vi "Read sequencia_ant.vi"(8 "error in (no error)":errorcluster, 11 "Opt_Selector in":refnum<class "Opt_Selector.lvclass">) -> (0 "error out":errorcluster, 2 "sequencia_ant":u16, 3 "Opt_Selector out":refnum<class "Opt_Selector.lvclass">)   [LabVIEW 2018, in "Opt_Selector.lvclass"]
uses:
  Opt_Selector.lvclass
  Opt_Selector.lvclass/Opt_Selector.ctl
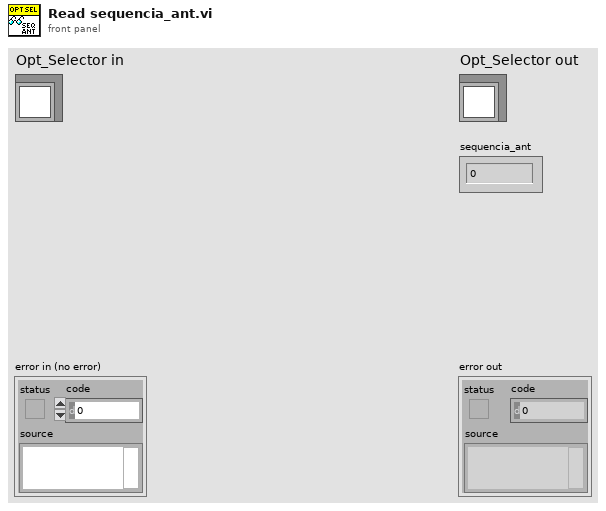
[diagram p1: front panel]
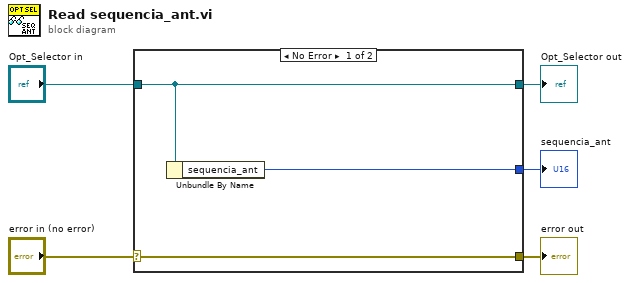
[diagram p0: block diagram]
diagram:
  n1 = case shown="No Error" "error in (no error)" {
    selector: "error in (no error)" -> [w8 w9]
    tunnel: [w8 w9] -> w4
    tunnel: [w7 w10] -> w2
    tunnel: "Opt_Selector in" -> [w7 w10]
    tunnel: [w6 _] -> w1
    frame No Error {
      n2 = Unbundle By Name(w7) -> ("sequencia_ant"=w6:u16)
    }
    frame Error {
    }
  }
  "error out" <- w4
  "Opt_Selector out" <- w2
  "sequencia_ant" <- w1
